vi "Write Data.vi"(8 "error in (no error)":errorcluster, 11 "file (use dialog)":path) -> (0 "error out":errorcluster)   [LabVIEW 2018]
uses:
  Main/Main Refs.ctl
  Hardware/Tecan/Pump Config.ctl
  Main/Vacuum Specs.ctl
  Main/Timing Specs.ctl
  Main/Cartridges.ctl
  Main/Cartridge Status.ctl
  Main/Commands.ctl
  Lib/Time/Wells.ctl
  Lib/Time/Bottles.ctl
  Main/Process State.ctl
  Main/Vacuum Test.ctl
panel:
  in  "Main References":T1
  # "Tecan Pump"
  # "Vacuum"
  # "General"
  # "Timing"
  # "Protocol"
  # "Zaber"
  # "NFC Reader 1"
  # "NFC  Reader 2"
  # "NFC Reader 3"
  # "NFC Reader 4"
  # "System"
  # "Cartridge Utitlies"
  # "Wells"
  # "times"
  # "from"
  # "State Machine"
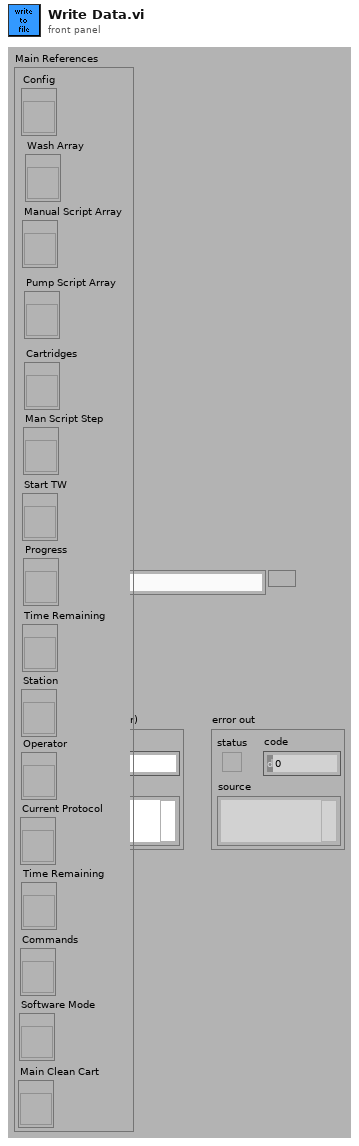
[diagram p1: front panel]
types:
  T1 = typedef "Main Refs.ctl" = cluster{"Config":refnum<vi>, "Wash Array":refnum<vi>, "Manual Script Array":refnum<vi>, "Pump Script Array":refnum<vi>, "Cartridges":refnum<vi>, "Man Script Step":refnum<vi>, "Start TW":refnum<vi>, "Progress":refnum<vi>, "Time Remaining":refnum<vi>, "Station":refnum<vi>, "Operator":refnum<vi>, "Current Protocol":refnum<vi>, "Time Remaining":refnum<vi>, "Commands":refnum<vi>, "Software Mode":refnum<vi>, "Main Clean Cart":refnum<vi>}
  T2 = enum16{"open", "replace", "create", "open or create", "replace or create", "replace or create with confirmation"}
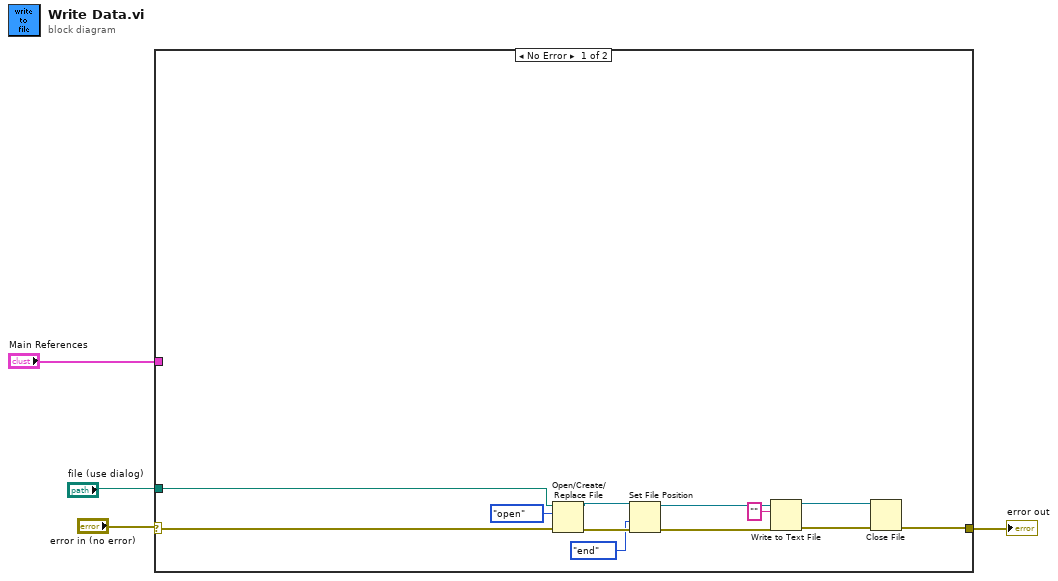
[diagram p0: block diagram]
diagram:
  n1 = case shown="No Error" "error in (no error)" {
    selector: "error in (no error)" -> [w16 w17]
    tunnel: [w13 w17] -> w3
    tunnel: "file (use dialog)" -> [w15 _]
    tunnel: "Main References" -> [_ _]
    frame No Error {
      n2 = Open/Create/Replace File(file path (use dialog)=w15, error in=w16, operation (0:open)=T2."open") -> (refnum out=w8:refnum<file>, error out=w10:errorcluster)  [unwired: 3 in, 1 out]
      n3 = Set File Position(refnum=w8, from (0:start)=enum16{"start", "end", "current"}."end", error in=w10) -> (refnum out=w7:refnum<file>, error out=w9:errorcluster)  [unwired: 1 in]
      n4 = Write to Text File(file (use dialog)=w7, text="", error in=w9) -> (refnum out=w12:refnum<file>, error out=w14:errorcluster)  [unwired: 1 in, 1 out]
      n5 = Close File(refnum=w12, error in=w14) -> (error out=w13:errorcluster)  [unwired: 1 out]
    }
    frame Error {
    }
  }
  "error out" <- w3
